vi "Send to CS.vi"(8 "error in (no error)":errorcluster, 10 "String to write":string, 11 "QCS in":refnum<class "QCS.lvclass">) -> (0 "error out":errorcluster, 3 "QCS out":refnum<class "QCS.lvclass">)   [LabVIEW 2013, in "QCS.lvclass"]
uses:
  Lib.llb/QCS.lvclass
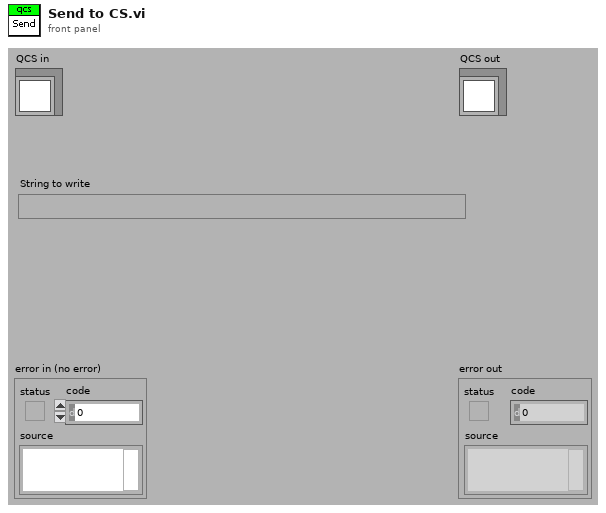
[diagram p1: front panel]
types:
  T1 = typedef "CS Data.ctl" = cluster{"Range":u8, "Current":dbl, "Current (string)":string, "On?":bool, "G?":bool, "I?":bool, "Err?":bool}
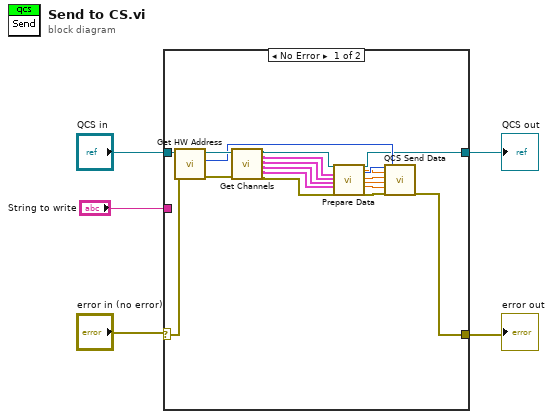
[diagram p0: block diagram]
diagram:
  n1 = case shown="No Error" "error in (no error)" {
    selector: "error in (no error)" -> [w23 w26]
    tunnel: [w13 w26] -> w4
    tunnel: [w6 w25] -> w3
    tunnel: "QCS in" -> [w24 w25]
    tunnel: "String to write" -> [_ _]
    frame No Error {
      n2 = call-dynamic "Get HW Address.vi"("error in (no error)"=w23, "CS.lvclass in"=w24) -> ("error out"=w16:errorcluster, "HW Address"=w15:u32, "CS.lvclass out"=w17:refnum<class "QCS.lvclass">)  [unwired: 7 in]
      n3 = call-dynamic "Get Channels.vi"("CS.lvclass in"=w17, "error in (no error)"=w16) -> ("CS.lvclass out"=w7:refnum<class "QCS.lvclass">, "I0"=w18:T1, "I1"=w19:T1, "I2"=w20:T1, "I3"=w21:T1, "error out"=w22:errorcluster)  [unwired: 12 in]
      n4 = call-dynamic "Prepare Data.vi"("CS in"=w7, "I0"=w18, "I1"=w19, "I2"=w20, "I3"=w21, "error in (no error)"=w22) -> ("Range bits"=w12:u32, "CS out"=w6:refnum<class "QCS.lvclass">, "V Out 0"=w11:dbl, "V Out 1"=w10:dbl, "V Out 2"=w9:dbl, "V Out 3"=w8:dbl, "error out"=w14:errorcluster)  [unwired: 15 in]
      n5 = call "QCS Send Data.vi"("Range bits"=w12, "V Out 0"=w11, "V Out 1"=w10, "V Out 2"=w9, "V Out 3"=w8, "error in (no error)"=w14, "HW Address"=w15) -> ("error out"=w13:errorcluster)  [unwired: 11 in, 1 out]
    }
    frame Error {
    }
  }
  "error out" <- w4
  "QCS out" <- w3
